vi "writeToXML.vi"(8 "error in (no error)":errorcluster, 10 "ClassLabel":string, 11 "DifftrackStatus in":refnum<class "DifftrackStatus.lvclass">) -> (0 "error out":errorcluster, 2 "XML out":string, 3 "DifftrackStatus out":refnum<class "DifftrackStatus.lvclass">)   [LabVIEW 2014, in "TCSDataDefinitions.lvlib" / "TCSPublicStatus.lvlib" / "PointingPositions.lvlib" / "DifftrackStatus.lvclass"]
uses:
  DifftrackStatus.lvclass
  <userlib>/Common/UnitsAndXML/FlattenItemWithUnitToXML/FlattenAngularVelocityToXML/AngularVelocityUnit.ctl
  DifftrackStatus.lvclass/DifftrackStatus.ctl
  <userlib>/Common/XML/XMLGenerator/XMLGenerator.lvclass
  <userlib>/Common/UnitsAndXML/UnitsAndXML.lvlib
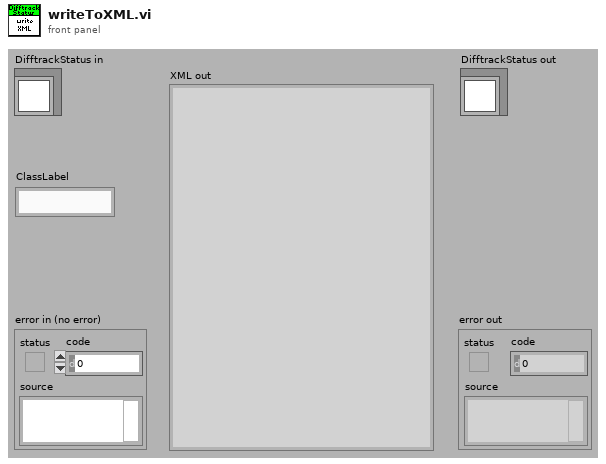
[diagram p1: front panel]
types:
  T1 = typedef "UnitsAndXML.lvlib/AngularVelocityUnit.ctl" = enum16{"\"/a", "deg/s", "\"/s"}
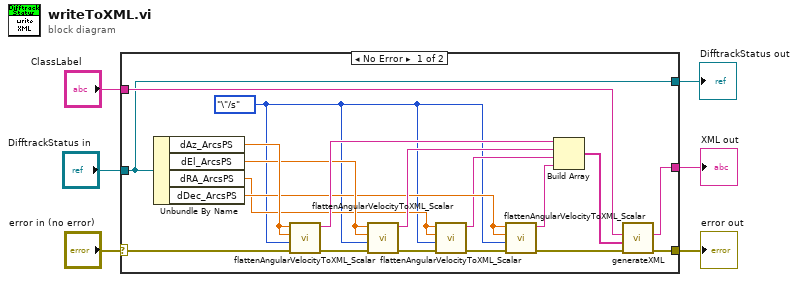
[diagram p0: block diagram]
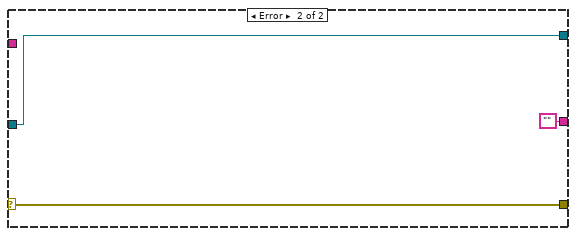
[diagram p2: hidden frame]
diagram:
  n1 = case shown="No Error" "error in (no error)" {
    selector: "error in (no error)" -> [w22 w28]
    tunnel: [w24 w28] -> w5
    tunnel: [w8 w27] -> w3
    tunnel: "DifftrackStatus in" -> [w8 w27]
    tunnel: "ClassLabel" -> [w23 _]
    tunnel: [w14 ""] -> w1
    frame No Error {
      w9 = AngularVelocityUnit."\"/s" ("angularVelocityUnitInXML")
      n2 = Unbundle By Name(w8) -> ("dAz_ArcsPS"=w20:dbl[unit], "dEl_ArcsPS"=w18:dbl[unit], "dRA_ArcsPS"=w11:dbl[unit], "dDec_ArcsPS"=w15:dbl[unit])
      n3 = call <userlib>:"flattenAngularVelocityToXML_Scalar.vi"("error in (no error)"=w22, "angularVelocityUnitInXML"=w9, "anuglarVelocityAgain"=w20, "angularVelocity"=w20) -> ("error out"=w19:errorcluster, "xmlString"=w21:string)  [unwired: 6 in]
      n4 = call <userlib>:"flattenAngularVelocityToXML_Scalar.vi"("error in (no error)"=w19, "angularVelocityUnitInXML"=w9, "anuglarVelocityAgain"=w18, "angularVelocity"=w18) -> ("error out"=w13:errorcluster, "xmlString"=w17:string)  [unwired: 6 in]
      n5 = call <userlib>:"flattenAngularVelocityToXML_Scalar.vi"("error in (no error)"=w13, "angularVelocityUnitInXML"=w9, "anuglarVelocityAgain"=w11, "angularVelocity"=w11) -> ("error out"=w12:errorcluster, "xmlString"=w10:string)  [unwired: 6 in]
      n6 = call <userlib>:"flattenAngularVelocityToXML_Scalar.vi"("error in (no error)"=w12, "angularVelocityUnitInXML"=w9, "anuglarVelocityAgain"=w15, "angularVelocity"=w15) -> ("error out"=w7:errorcluster, "xmlString"=w16:string)  [unwired: 6 in]
      n7 = Build Array(w21, w17, w10, w16) -> (w25:string[])
      n8 = call <userlib>:"generateXML.vi"("error in"=w7, "childrenXML"=w25, "elementName"=w23) -> ("error out"=w24:errorcluster, "XML out"=w14:string)  [unwired: 6 in, 1 out]
    }
    frame Error {
    }
  }
  "error out" <- w5
  "XML out" <- w1
  "DifftrackStatus out" <- w3
